vi "Increment Framework Cycle.vi"(8 "error in (no error)":errorcluster, 11 "Framework in":refnum<class "Framework.lvclass">) -> (0 "error out":errorcluster, 3 "Framework out":refnum<class "Framework.lvclass">)   [LabVIEW 2017, in "DSF Core.lvlib" / "Framework.lvclass"]
uses:
  Framework.lvclass
  Framework.lvclass/Framework.ctl
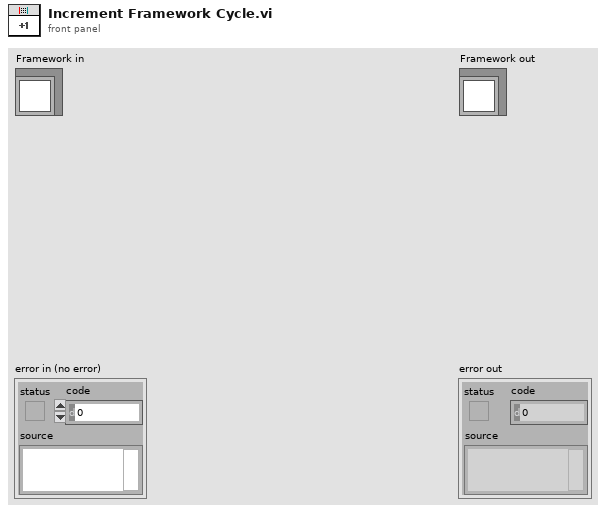
[diagram p1: front panel]
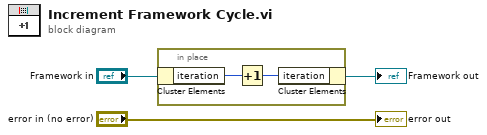
[diagram p0: block diagram]
diagram:
  n1 = in-place {
    n2 = in-place-cluster #1("Framework in") -> ("iteration"=w5:u64)
    n3 = Increment(x=w5) -> (x+1=w4:u64)
    n4 = in-place-cluster #1("iteration"=w4) -> (→"Framework out":refnum<class "Framework.lvclass">)
  }
  "error out" <- "error in (no error)"
